vi "Write SamplesPerCycle.vi"(8 "error in (no error)":errorcluster, 10 "SamplesPerCycle":u16, 11 "nCRD in":refnum<class "nCRD.lvclass">) -> (0 "error out":errorcluster, 3 "nCRD out":refnum<class "nCRD.lvclass">)   [LabVIEW 2013, in "nCRD.lvclass"]
uses:
  nCRD.lvclass
  nCRD.lvclass/nCRD.ctl
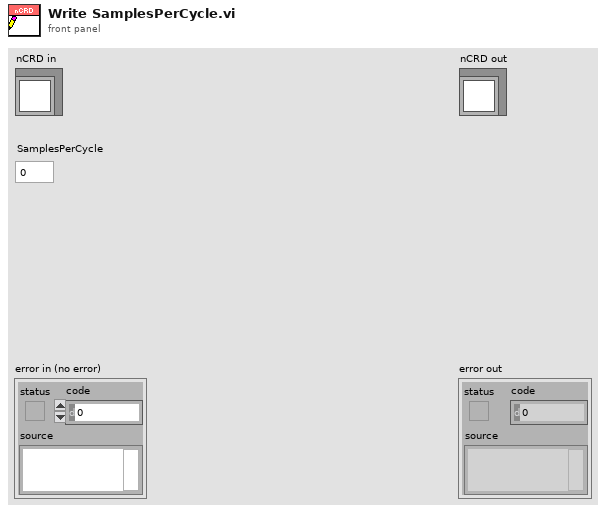
[diagram p1: front panel]
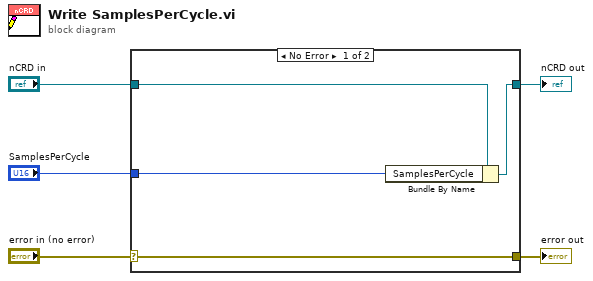
[diagram p0: block diagram]
diagram:
  n1 = case shown="No Error" "error in (no error)" {
    selector: "error in (no error)" -> [w9 w10]
    tunnel: [w9 w10] -> w4
    tunnel: [w7 w11] -> w2
    tunnel: "nCRD in" -> [w8 w11]
    tunnel: "SamplesPerCycle" -> [w6 _]
    frame No Error {
      n2 = Bundle By Name(cluster=w8, "SamplesPerCycle"=w6) -> (w7:refnum<class "nCRD.lvclass">)
    }
    frame Error {
    }
  }
  "error out" <- w4
  "nCRD out" <- w2
